vi "PCO_SetDoubleImageMode.vi"(8 "error in (no error)":errorcluster {"code" format="%x"}, 10 "wDoubleImage":u16(ring) items=["OFF", "ON"], 11 "ph":u64) -> (0 "error out":errorcluster {"code" format="%x"}, 2 "ErrorMessage":i32 format="%x", 3 "ph out":u64)   [LabVIEW 2019, in "SDK.lvlib" / "ImageSensor.lvlib"]
doc: "<b>Description:</b>\nThis function does set the double image operating mode. Cameras with activated double image mode readout two exposures separated by a short interleaving time. The resulting double image is transferred as one frame that means the two images resulting from the two / double exposures are stitched together as one and are counted as one.\nThus the buffer size of all allocated buffers has to be doubled. The first half of the buffer will be filled with the first exposed frame (image A). The second exposed frame (image B) will be transferred to the second half of the buffer.\nInvalid values result in a failure response message.\nThe command will be rejected, if Recording State is [run], see PCO_GetRecordingState.\n\n<b>Supported camera type:</b>\nAll cameras\n\n<b>Descriptor dependency:</b>\nwDoubleImageDESC"
uses:
  ImageSensor.lvlib
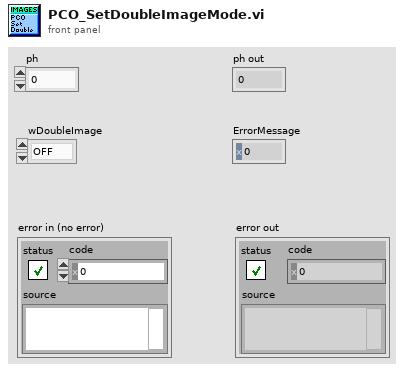
[diagram p1: front panel]
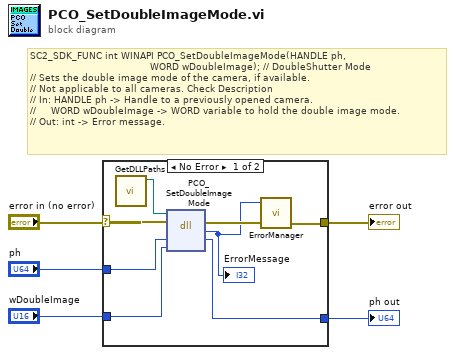
[diagram p0: block diagram]
diagram:
  # "SC2_SDK_FUNC int WINAPI PCO_SetDoubleImageMode(HANDLE ph,\n                                        WORD wDoubleImage); // DoubleShutter Mode\n// Sets the double image mode of the camera, if available.\n// Not applicable to all cameras. Check Description\n// In: HANDLE ph -> Handle to a previously opened camera.\n//     WORD wDoubleImage -> WORD variable to hold the double image mode.\n// Out: int -> Error message."
  n1 = case shown="No Error" "error in (no error)" {
    selector: "error in (no error)" -> [w10 w15]
    tunnel: "ph" -> [w13 w14]
    tunnel: [w12 w14] -> w4
    tunnel: "wDoubleImage" -> [w11 _]
    tunnel: [w8 w15] -> w2
    frame No Error {
      n2 = call "GetDLLPaths.vi"() -> ("SC2_Cam_Path"=w6:path)  [unwired: 9 in, 2 out]
      n3 = dll-call lib="?" fn="PCO_SetDoubleImageMode"(path in=w6, error in=w10, "ph"=w13, "wDoubleImage"=w11) -> (error out=w9:errorcluster, "return type"=w7:i32, "ph"=w12:u64)  [unwired: 2 in, 1 out]
      "ErrorMessage" <- w7
      n4 = call "ErrorManager.vi"("error in (no error)"=w9, "error code"=w7) -> ("error out"=w8:errorcluster)  [unwired: 3 in]
    }
    frame Error {
    }
  }
  "ph out" <- w4
  "error out" <- w2
